vi "Display Mode.vi"(8 "error in (no error)":errorcluster, 10 "Display Mode":bool, 11 "UI - Controller -- Interface in":refnum<class "UI - Controller -- Interface.lvclass">) -> (0 "error out":errorcluster, 3 "UI - Controller -- Interface out":refnum<class "UI - Controller -- Interface.lvclass">)   [LabVIEW 2022 SP3, in "UI - Controller -- Interface.lvlib" / "UI - Controller -- Interface.lvclass"]
uses:
  UI - Controller -- Interface.lvclass
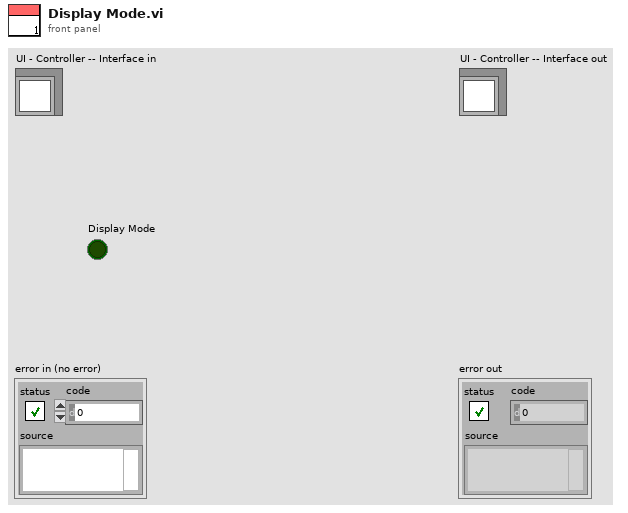
[diagram p1: front panel]
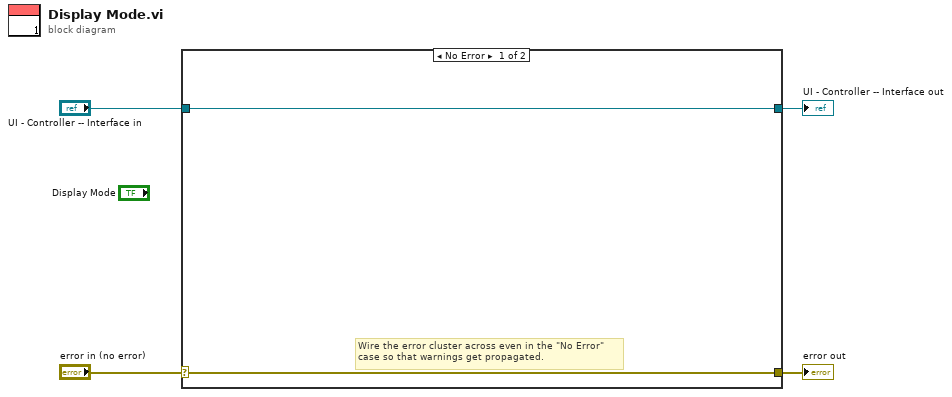
[diagram p0: block diagram]
diagram:
  n1 = case shown="No Error" "error in (no error)" {
    selector: "error in (no error)" -> [w5 w8]
    tunnel: [w5 w8] -> w3
    tunnel: [w6 w7] -> w1
    tunnel: "UI - Controller -- Interface in" -> [w6 w7]
    frame No Error {
      # "Wire the error cluster across even in the \"No Error\"\ncase so that warnings get propagated."
    }
    frame Error {
    }
  }
  "error out" <- w3
  "UI - Controller -- Interface out" <- w1
